vi "Write Config Ref.vi"(8 "error in (no error)":errorcluster, 11 "Configuration File In":refnum<class "Configuration.lvclass">) -> (0 "error out":errorcluster, 3 "Configuration File Out":refnum<class "Configuration.lvclass">, 10 "Reference":variant)   [LabVIEW 2020, in "Configuration.lvclass"]
doc: "For the configuration interface to work, the class implementing the interface needs to save the reference to the implementation in the class attributes. This is an accessor for that attribute which must be implemented by the class."
uses:
  Configuration.lvclass
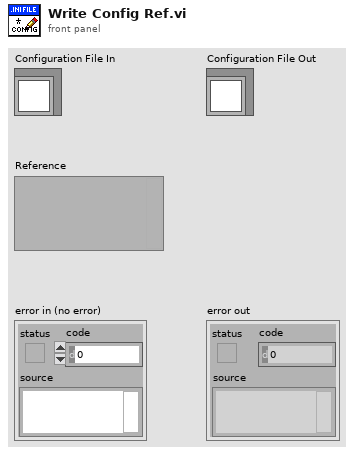
[diagram p1: front panel]
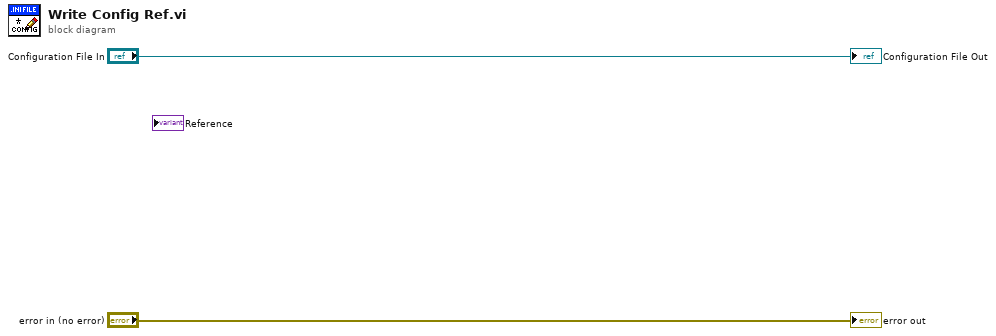
[diagram p0: block diagram]
diagram:
  "error out" <- "error in (no error)"
  "Configuration File Out" <- "Configuration File In"
